vi "Get_Error_Status.vi"(5 "Device Number":T1, 7 "Update":bool, 8 "error in":errorcluster) -> (0 "error out":errorcluster)   [LabVIEW 2016]
doc: "This navX VI returns the velocity and displacement of the navX. This VI is only supported on firmware virsions newer than 2.2.xxx."
uses:
  _TypeDefs/FRIC_navX_DeviceNumbersTypeDef.ctl
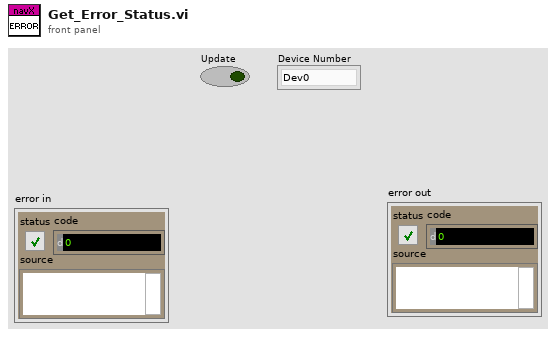
[diagram p1: front panel]
types:
  T1 = typedef "FRIC_navX_DeviceNumbersTypeDef.ctl" = enum16{"Dev0", "Dev1", "Dev2", "Dev3"}
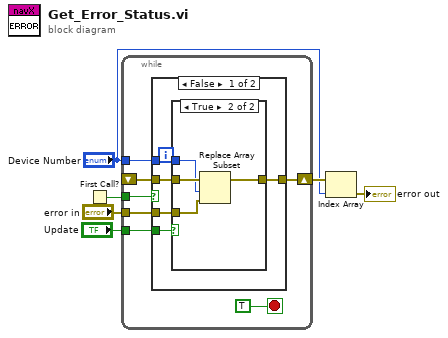
[diagram p0: block diagram]
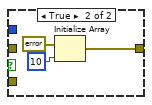
[diagram p3: hidden frame]
diagram:
  n1 = First Call?() -> (First Call?: T/F=w3:bool)
  n2 = while {
    shift-right: [w13] -> w5
    shift-left: _ -> [w11]
    tunnel: "Update" -> [w10]
    tunnel: "Device Number" -> [w9]
    tunnel: w3 -> [w8]
    tunnel: "error in" -> [w7]
    stop <- TRUE stop-if-true
    n3 = case shown="False" w8 {
      tunnel: [w18 w25] -> w13
      tunnel: w11 -> [w17 _]
      tunnel: w10 -> [w15 _]
      tunnel: w9 -> [w16 _]
      tunnel: w7 -> [w14 _]
      frame False {
        n4 = case shown="True" w15 {
          tunnel: [w19 w22] -> w18
          tunnel: w17 -> [w19 w23]
          tunnel: w16 -> [_ w21]
          tunnel: w14 -> [_ w20]
          frame False {
          }
          frame True {
            n5 = Replace Array Subset(array=w23, new element=w20, index=w21) -> (w22:errorcluster[])
          }
        }
      }
      frame True {
        n6 = Initialize Array(errorcluster {"status"=FALSE, "code"=0, "source"=""} ("error"), 10 ("dimension size")) -> (w25:errorcluster[])
      }
    }
  }
  n7 = Index Array(array=w5, index="Device Number") -> (element=→"error out":errorcluster)
